vi "CCDSetAndGetFitParams.vi"   [LabVIEW 2023]
uses:
  <vilib>/addons/_JKI Toolkits/Caraya/classes/Test/Test.lvclass
  <vilib>/addons/_JKI Toolkits/Caraya/classes/Assert/Assert.lvclass
  Source/Classes/CCD/CCD.lvclass
  <vilib>/addons/_JKI Toolkits/Caraya/classes/Assert/Assert Not Error.vi
  <vilib>/addons/_JKI Toolkits/Caraya/classes/Assert/Assert Equal Value and Type_Variant.vi
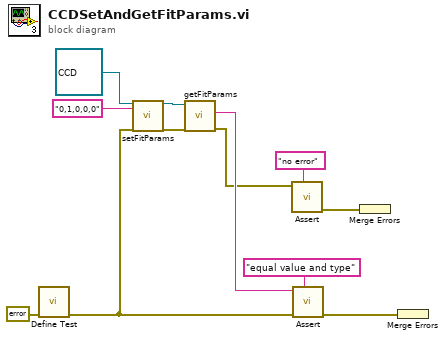
[diagram p0: block diagram]
diagram:
  n1 = call <vilib>:"Define Test.vi"("error in (no error)"=errorcluster {"status"=FALSE, "code"=0, "source"=""}) -> ("error out"=w6:errorcluster)  [unwired: 9 in, 1 out]
  n2 = call "setFitParams.vi"("CCD in"=refnum<class "CCD.lvclass"> refnum, "fit parameters"="0,1,0,0,0", "error in (no error)"=w6) -> ("CCD out"=w5:refnum<class "CCD.lvclass">, "error out"=w2:errorcluster)  [unwired: 11 in, 4 out]
  n3 = call "getFitParams.vi"("error in (no error)"=w2, "CCD in"=w5) -> ("error out"=w1:errorcluster, "fit parameters"=w3:string)  [unwired: 7 in, 1 out]
  n4 = call-poly <vilib>:"Assert.vi"("Label"="no error" ("Label (VI Title)"), "Not Error?"=w1) -> ("error out"=w8:errorcluster)  [unwired: 8 in, 1 out]
  n5 = call-poly <vilib>:"Assert.vi"("Label"="equal value and type" ("Label (VI Title)"), "error in (no error)"=w6, "X"=w3) -> ("error out"=w11:errorcluster)  [unwired: 7 in, 1 out]
  n6 = Merge Errors(w8) -> ()  [unwired: 1 out]
  n7 = Merge Errors(w11) -> ()  [unwired: 1 out]
